vi "Combine Particles.vi"(11 "Good particles in":T1(array[cluster])) -> ()   [LabVIEW 2014]
panel:
  out "_| Particles":T1(array[cluster])
  out "Partners":T1(array[cluster])
  out "Partner Found?":bool[](array[boolean])
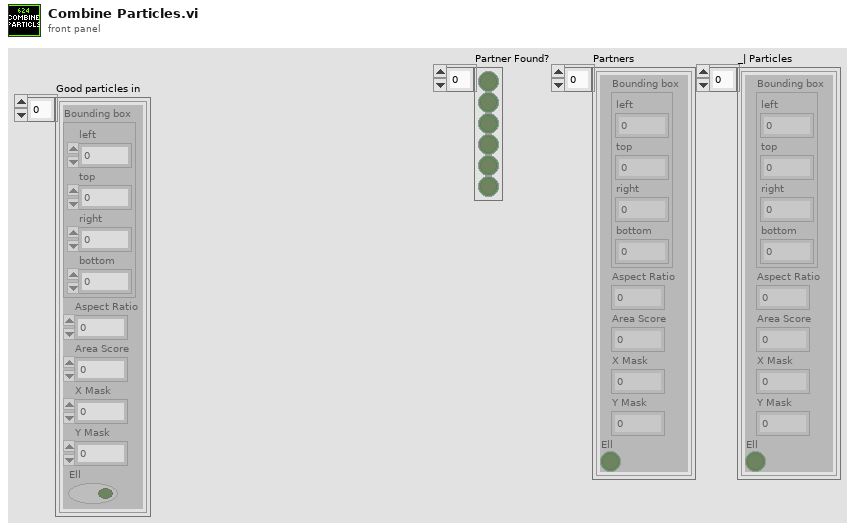
[diagram p1: front panel]
types:
  T1 = cluster{"Bounding box":cluster{"left":dbl, "top":dbl, "right":dbl, "bottom":dbl}, "Aspect Ratio":dbl, "Area Score":dbl, "X Mask":dbl, "Y Mask":dbl, "Ell":bool}[]
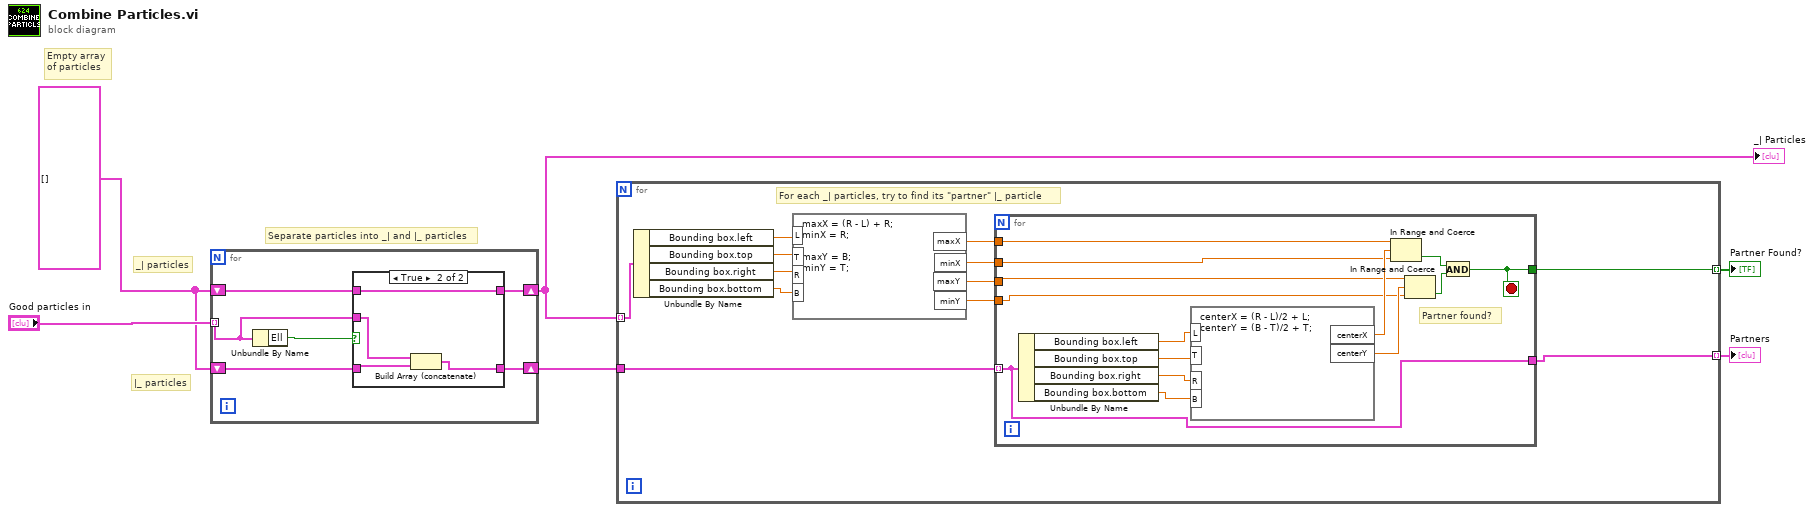
[diagram p0: block diagram]
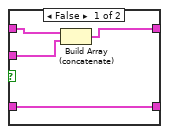
[diagram p2: hidden frame]
diagram:
  w5 = T1 [] ("Good particles in")
  # "Separate particles into _| and |_ particles"
  # "|_ particles"
  # "_| particles"
  # "Empty array\nof particles"
  n1 = for {
    tunnel: "Good particles in" -> [w8] mode=indexing
    shift-right: [w9] -> w4
    shift-left: w5 -> [w11]
    shift-right: [w7] -> w3
    shift-left: w5 -> [w10]
    n2 = Unbundle By Name(w8) -> ("Ell"=w12:bool)
    n3 = case shown="True" w12 {
      tunnel: w11 -> [w16 w20]
      tunnel: w10 -> [w13 w18]
      tunnel: [w15 w20] -> w9
      tunnel: w8 -> [w14 w19]
      tunnel: [w13 w17] -> w7
      frame False {
        n4 = Build Array (concatenate)(w16, w14) -> (w15:T1)
      }
      frame True {
        n5 = Build Array (concatenate)(w19, w18) -> (w17:T1)
      }
    }
  }
  "_| Particles" <- w4
  n6 = for {
    tunnel: w4 -> [w31] mode=indexing
    tunnel: w3 -> [w32]
    tunnel: [w22] -> w2 mode=indexing
    tunnel: [w21] -> w1 mode=indexing
    # "For each _| particles, try to find its \"partner\" |_ particle"
    n7 = Unbundle By Name(w31) -> ("Bounding box.left"=w30:dbl, "Bounding box.top"=w29:dbl, "Bounding box.right"=w28:dbl, "Bounding box.bottom"=w27:dbl)
    n8 = formula code="maxX = (R - L) + R;\nminX = R;\n\nmaxY = B;\nminY = T;"("L"=w30, "T"=w29, "R"=w28, "B"=w27) -> ("maxX"=w26:dbl, "minX"=w25:dbl, "maxY"=w24:dbl, "minY"=w23:dbl)
    n9 = for {
      tunnel: w32 -> [w33] mode=indexing
      tunnel: w26 -> [w41]
      tunnel: w25 -> [w40]
      tunnel: w24 -> [w38]
      tunnel: w23 -> [w37]
      tunnel: [w34] -> w22
      tunnel: [w33] -> w21
      stop <- w34 stop-if-true
      # "Partner found?"
      n10 = Unbundle By Name(w33) -> ("Bounding box.left"=w46:dbl, "Bounding box.top"=w45:dbl, "Bounding box.right"=w44:dbl, "Bounding box.bottom"=w43:dbl)
      n11 = formula code="centerX = (R - L)/2 + L;\ncenterY = (B - T)/2 + T;"("L"=w46, "T"=w45, "R"=w44, "B"=w43) -> ("centerX"=w42:dbl, "centerY"=w39:dbl)
      n12 = In Range and Coerce(upper limit=w41, x=w42, lower limit=w40) -> (In Range?=w35:bool)  [unwired: 1 out]
      n13 = In Range and Coerce(upper limit=w38, x=w39, lower limit=w37) -> (In Range?=w36:bool)  [unwired: 1 out]
      n14 = And(x=w35, y=w36) -> (x .and. y?=w34:bool)
    }
  }
  "Partner Found?" <- w2
  "Partners" <- w1
